vi "ADIS16448 Loop.vi"(8 "error in":errorcluster) -> ()   [LabVIEW 2019]
uses:
  Typedef/ADIS16448 Device Reference.ctl
  Typedef/ADIS16448 Hardware Configuration.ctl
  <vilib>/Rock Robotics/WPI/SPI/WPI_SPIMode.ctl
  <vilib>/Rock Robotics/SystemInterfaces/DIO/FPGA_DIOChannel.ctl
  <vilib>/Rock Robotics/SystemInterfaces/spilib/spi_bus.ctl
  Typedef/ADIS16448 Status.ctl
  Typedef/ADIS16448 Data.ctl
  Typedef/ADIS16448 Process.ctl
  Typedef/ADIS16448 Command Type.ctl
  <vilib>/Rock Robotics/SystemInterfaces/CounterEncoderSourceConvertion/FPGA_CounterEncoderSourceConvertionLVSourceType.ctl
  <vilib>/Rock Robotics/SystemInterfaces/DIO/FPGA_DIODigitalSourceChannel.ctl
  <vilib>/Rock Robotics/SystemInterfaces/AnalogTrigger/FPGA_AnalogTriggerIndex.ctl
  <vilib>/Rock Robotics/SystemInterfaces/AnalogTrigger/FPGA_AnalogTriggerOutType.ctl
  <vilib>/Rock Robotics/WPI/SPI/WPI_SPIDevRef.ctl
  Typedef/ADIS16448 Register.ctl
  <vilib>/Rock Robotics/WPI/Counter/WPI_CounterDigitalInputToDigitalSource.vi
  <vilib>/ptbypt/NI_PtbyPt.lvlib
panel:
  in  "Calibration Time":i32
  in  "element":T1
  in  "ADIS16448DevRef":T2={"DevStatus"={"status"=FALSE, "code"=0, "source"=""}, "Hardware Config"={"SPI Clock Rate (Hz)"=1000000.0, "IMU SPI Mode (3)"=enum."Mode 3 (Clk Idle High,Sample on Trailing)", "IMU Reset Pin"=enum."SPI Port CS2", "IMU SPI Bus"=enum."SPI On-Board, CS0", "IMU Data Ready Pin"=enum."SPI Port CS1", "Stall Config"={"Pow2BytesPerRead"=255, "StallTicks"=640, "CsToSclkTicks"=5}, "IMU Status LED Pin"=enum."DIO MXP 9"}, "Calibration Complete"=refnum, "Status FIFO"=refnum, "Last Value Reference"=refnum, "Sychronous Process VI"=refnum, "Cmd FIFO"=refnum, "Source"={"DevStatus"={"status"=FALSE, "code"=0, "source"=""}, "AnalogTriggerMode?"=FALSE, "DigitalMode"={"DIO Channel"=enum."Disabled"}, "AnalogTriggerMode"={"AnalogTriggerIndex"=enum."Trig 0", "OutputType"=enum."InWindow"}}, "Data FIFO"=refnum, "IMU Status LED Pin"=enum."DIO MXP 9", "Calibration Time"=5}
  in  "Main Name":string
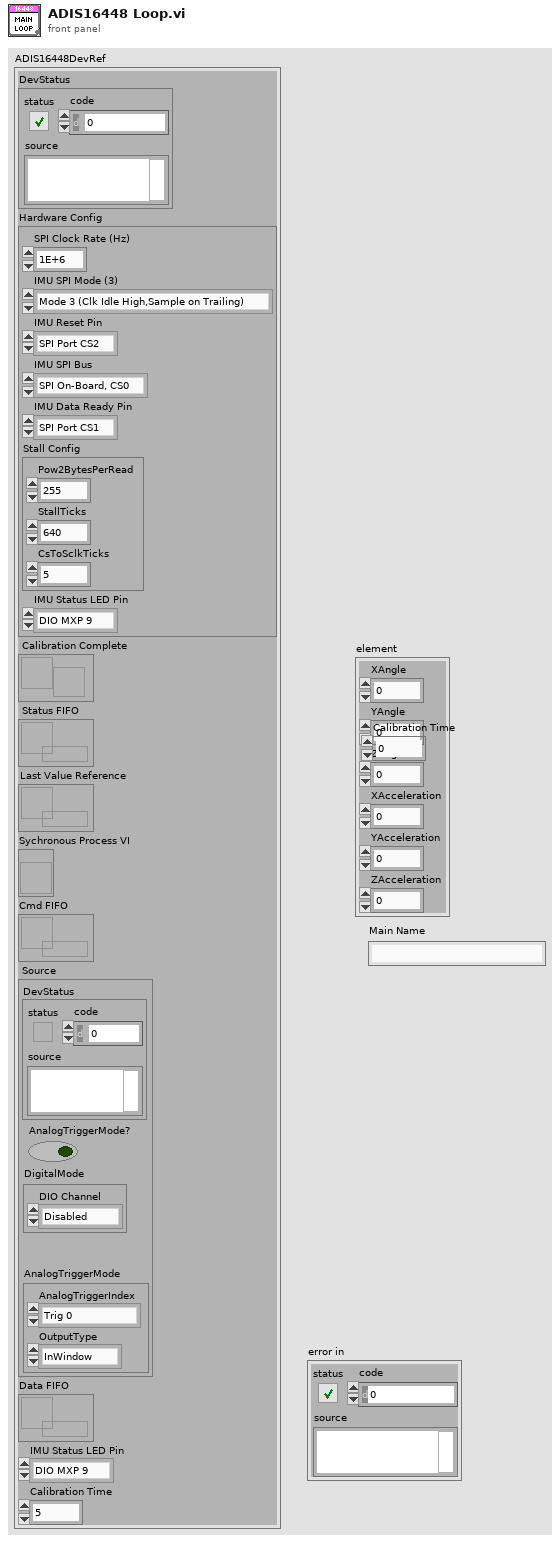
[diagram p1: front panel]
types:
  T1 = typedef "ADIS16448 Data.ctl" = cluster{"XAngle":dbl, "YAngle":dbl, "ZAngle":dbl, "XAcceleration":dbl, "YAcceleration":dbl, "ZAcceleration":dbl}
  T2 = typedef "ADIS16448 Device Reference.ctl" = cluster{"DevStatus":errorcluster, "Hardware Config":T3, "Calibration Complete":refnum<notifier>, "Status FIFO":refnum<k33>, "Last Value Reference":refnum<data-value>, "Sychronous Process VI":T7, "Cmd FIFO":refnum<k33>, "Source":T8, "Data FIFO":refnum<k33>, "IMU Status LED Pin":T5, "Calibration Time":u32}
  T3 = typedef "ADIS16448 Hardware Configuration.ctl" = cluster{"SPI Clock Rate (Hz)":dbl, "IMU SPI Mode (3)":T4, "IMU Reset Pin":T5, "IMU SPI Bus":T6, "IMU Data Ready Pin":T5, "Stall Config":cluster{"Pow2BytesPerRead":u8, "StallTicks":u16, "CsToSclkTicks":u8}, "IMU Status LED Pin":T5}
  T4 = typedef "WPI_SPIMode.ctl" = enum16{"Mode 0 (Clk Idle Low,Sample on Leading)", "Mode 1 (Clk Idle Low,Sample on Trailing)", "Mode 2 (Clk Idle High,Sample on Leading)", "Mode 3 (Clk Idle High,Sample on Trailing)"}
  T5 = typedef "FPGA_DIOChannel.ctl" = enum8{"DIO 0", "DIO 1", "DIO 2", "DIO 3", "DIO 4", "DIO 5", "DIO 6", "DIO 7", "DIO 8", "DIO 9", "DIO MXP 0", "DIO MXP 1", "DIO MXP 2", "DIO MXP 3", "DIO MXP 4", "DIO MXP 5", "DIO MXP 6", "DIO MXP 7", "DIO MXP 8", "DIO MXP 9", "DIO MXP 10", "DIO MXP 11", "DIO MXP 12", "DIO MXP 13", "DIO MXP 14", "DIO MXP 15", "SPI Port CS1", "SPI Port CS2", "SPI Port CS3", "SPI Port MISO", "SPI Port MOSI", "Invalid"}
  T6 = typedef "spi_bus.ctl" = enum16{"SPI On-Board, CS0", "SPI On-Board, CS1", "SPI On-Board, CS2", "SPI On-Board, CS3", "SPI MXP", "Invalid"}
  T7 = typedef "ADIS16448 Process.ctl" = refnum<vi>
  T8 = typedef "FPGA_CounterEncoderSourceConvertionLVSourceType.ctl" = cluster{"DevStatus":errorcluster, "AnalogTriggerMode?":bool, "DigitalMode":cluster{"DIO Channel":T9}, "AnalogTriggerMode":cluster{"AnalogTriggerIndex":T10, "OutputType":T11}}
  T9 = typedef "FPGA_DIODigitalSourceChannel.ctl" = enum8{"DIO 0", "DIO 1", "DIO 2", "DIO 3", "DIO 4", "DIO 5", "DIO 6", "DIO 7", "DIO 8", "DIO 9", "DIO MXP 0", "DIO MXP 1", "DIO MXP 2", "DIO MXP 3", "DIO MXP 4", "DIO MXP 5", "DIO MXP 6", "DIO MXP 7", "DIO MXP 8", "DIO MXP 9", "DIO MXP 10", "DIO MXP 11", "DIO MXP 12", "DIO MXP 13", "DIO MXP 14", "DIO MXP 15", "SPI Port CS1", "SPI Port CS2", "SPI Port CS3", "SPI Port MISO", "SPI Port MOSI", "Disabled"}
  T10 = typedef "FPGA_AnalogTriggerIndex.ctl" = enum8{"Trig 0", "Trig 1", "Trig 2", "Trig 3", "Trig 4", "Trig 5", "Trig 6", "Trig 7", "Invalid"}
  T11 = typedef "FPGA_AnalogTriggerOutType.ctl" = enum16{"InWindow", "TriggerState", "Rising", "Falling"}
  T12 = typedef "WPI_SPIDevRef.ctl" = cluster{"DevStatus":errorcluster, "Handle":i32, "SPI Bus":T6}
  T13 = cluster{"SPIDevRef":T12, "Data Counter":u16, "Reset":bool, "Digital Source":T8, "Bytes Per Sample":u32, "Data":dbl[], "ADIS16448DevRef":T2, "TimeStampPrev":u32, "Sensor to Robot Rotation":dbl[][], "AutoSPI Active?":bool, "Offsets":dbl[], "Offset Counter":i32, "Data Header":u8[], "Zero Byte Count":u8, "Running Offset":dbl[]}
  T14 = typedef "ADIS16448 Status.ctl" = cluster{"Calibrated?":bool, "IMU Detected?":bool}
  T15 = typedef "ADIS16448 Register.ctl" = u8
  T16 = typedef "ADIS16448 Command Type.ctl" = cluster{"Command":enum16{"None", "Reset", "Rewrite Config", "Start Recal", "Recalibrate", "Recal Complete", "Exit Auto SPI", "Start Auto SPI", "Configure Cal"}, "Data":u32}
  T17 = typedef "WPI_DigitalOutputDevRef.ctl" = cluster{"DIO Channel":T5, "DevStatus":errorcluster}
  T18 = typedef "WPI_DigitalInputDevRef.ctl" = cluster{"DevStatus":errorcluster, "DIO Channel":T5}
  T19 = cluster{"Pow2BytesPerRead":u8, "StallTicks":u16, "CsToSclkTicks":u8}
  T20 = enum16{"None", "Reset", "Rewrite Config", "Start Recal", "Recalibrate", "Recal Complete", "Exit Auto SPI", "Start Auto SPI", "Configure Cal"}
  T21 = enum32{"Bad", "Idle", "Run top level", "Running"}
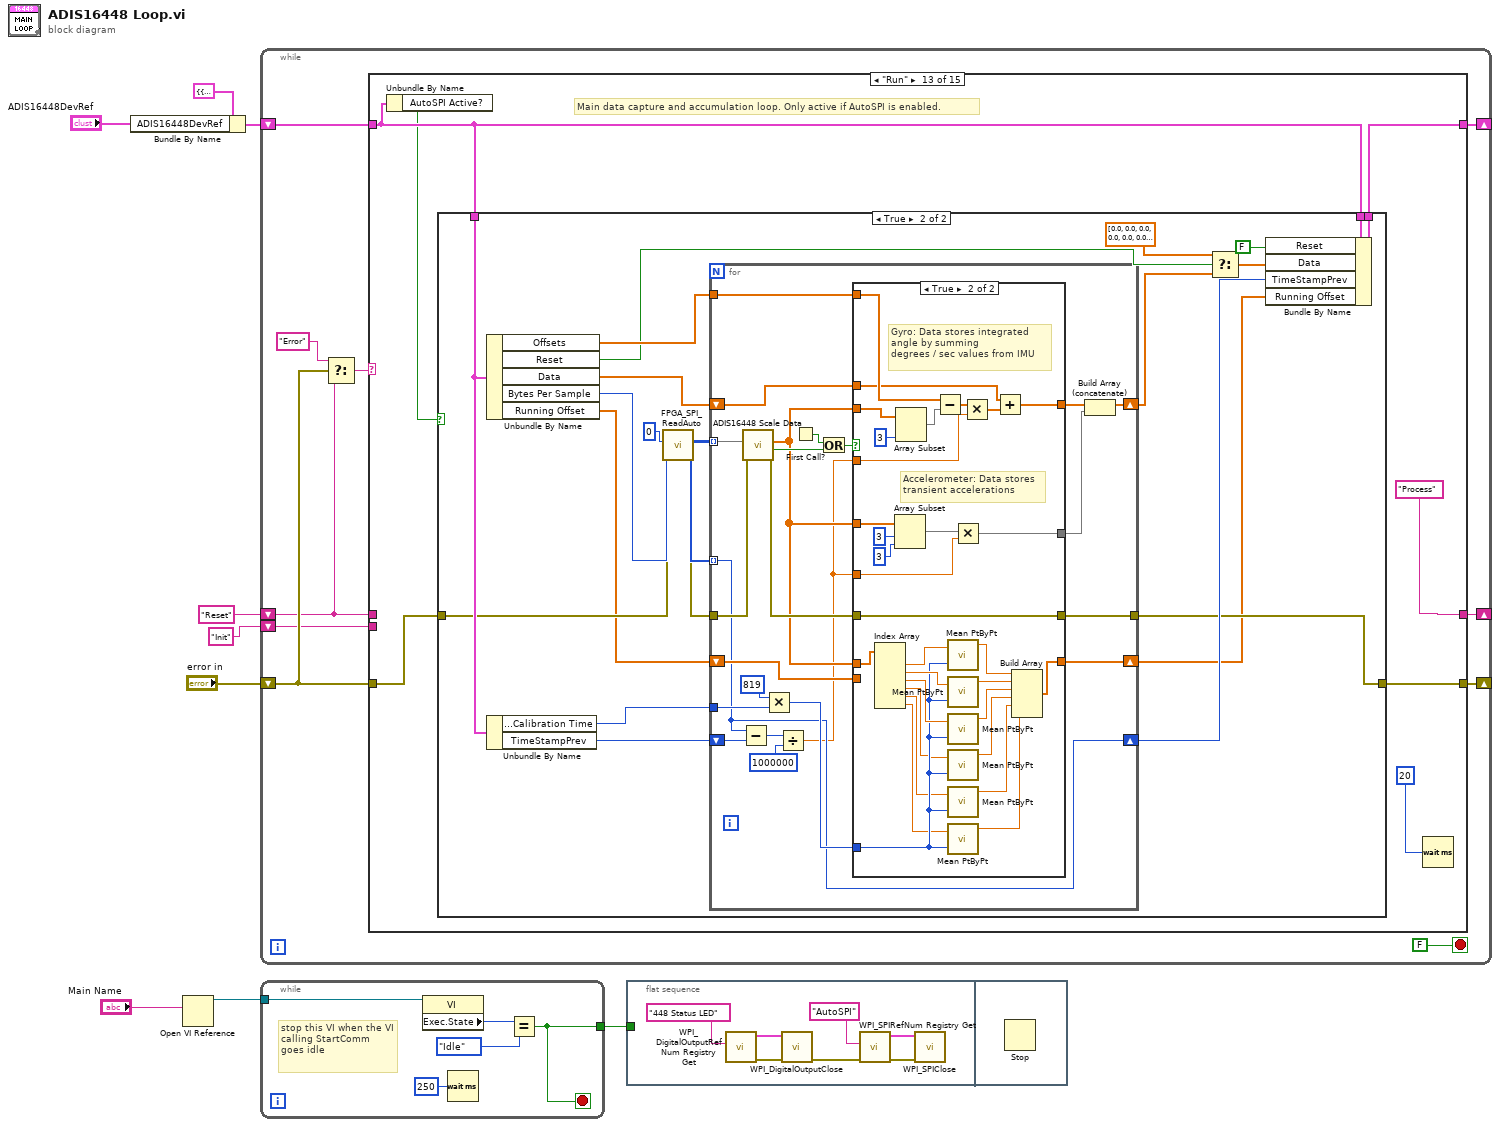
[diagram p0: block diagram]
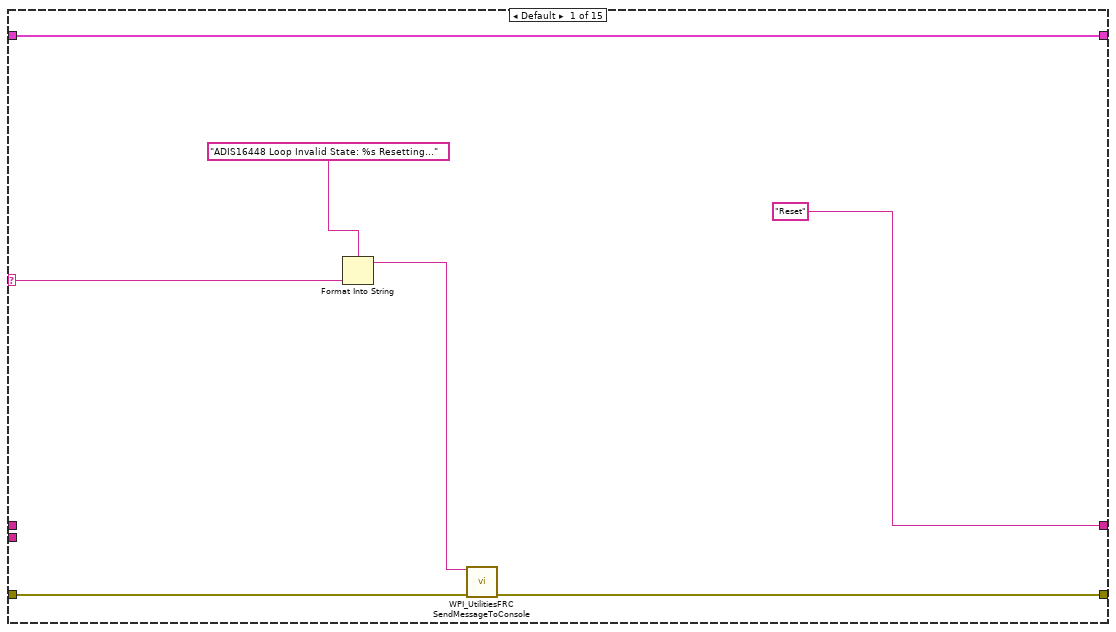
[diagram p2: hidden frame]
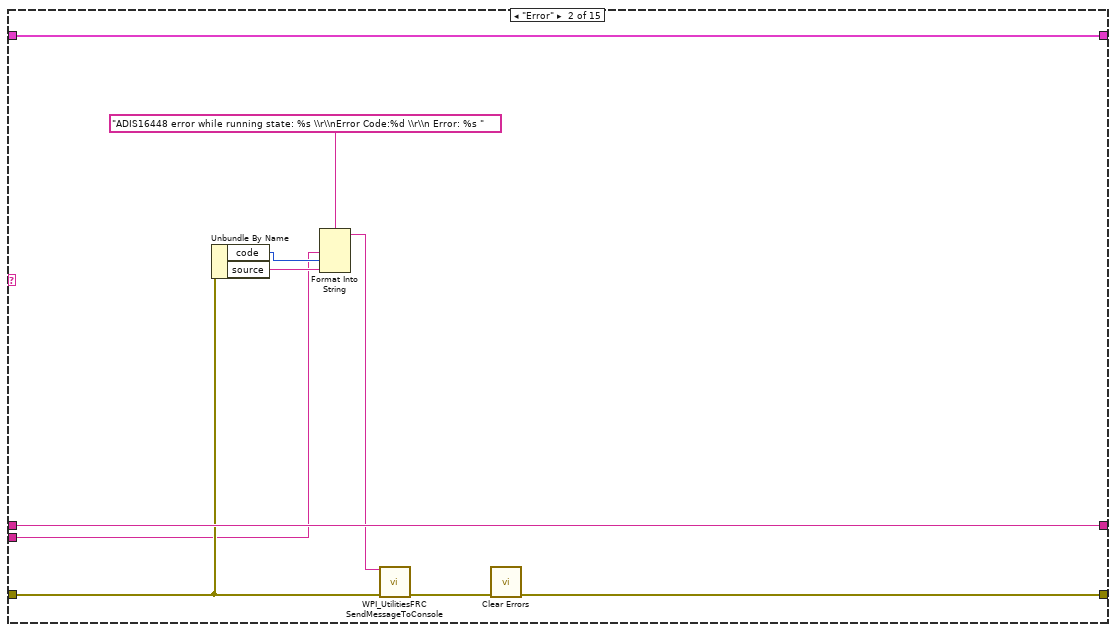
[diagram p3: hidden frame]
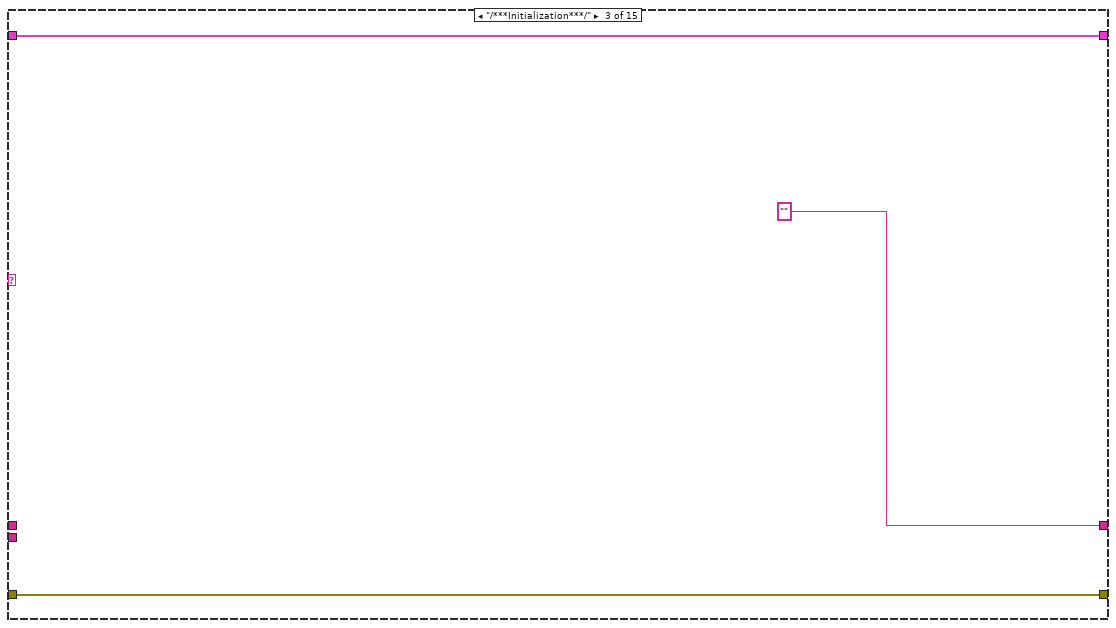
[diagram p4: hidden frame]
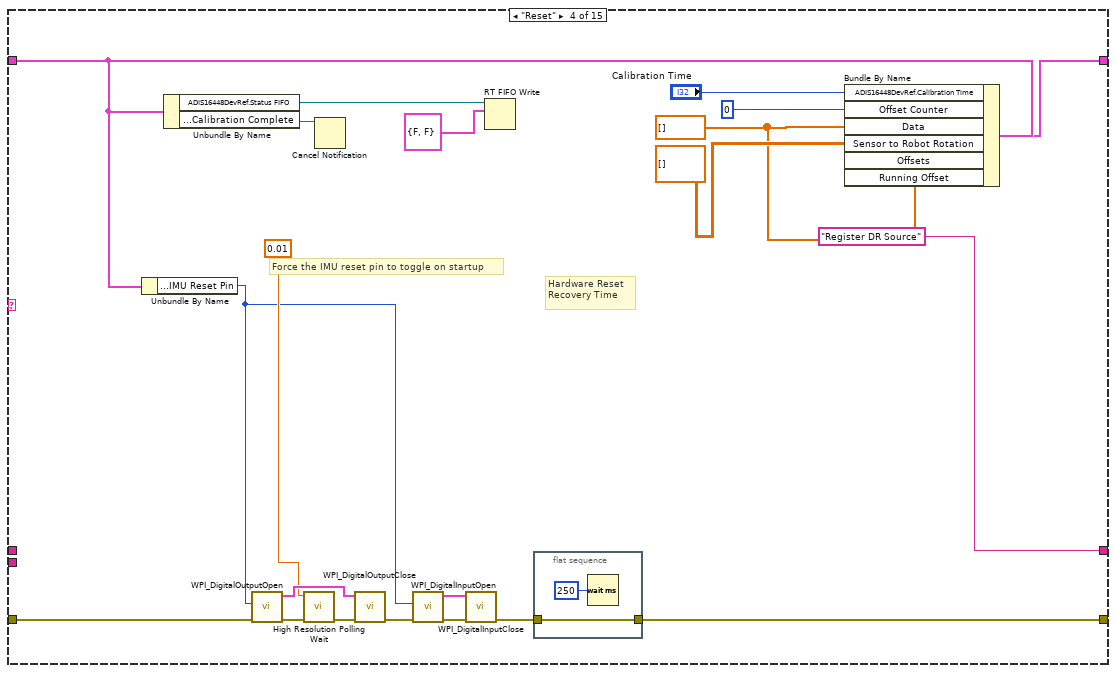
[diagram p5: hidden frame]
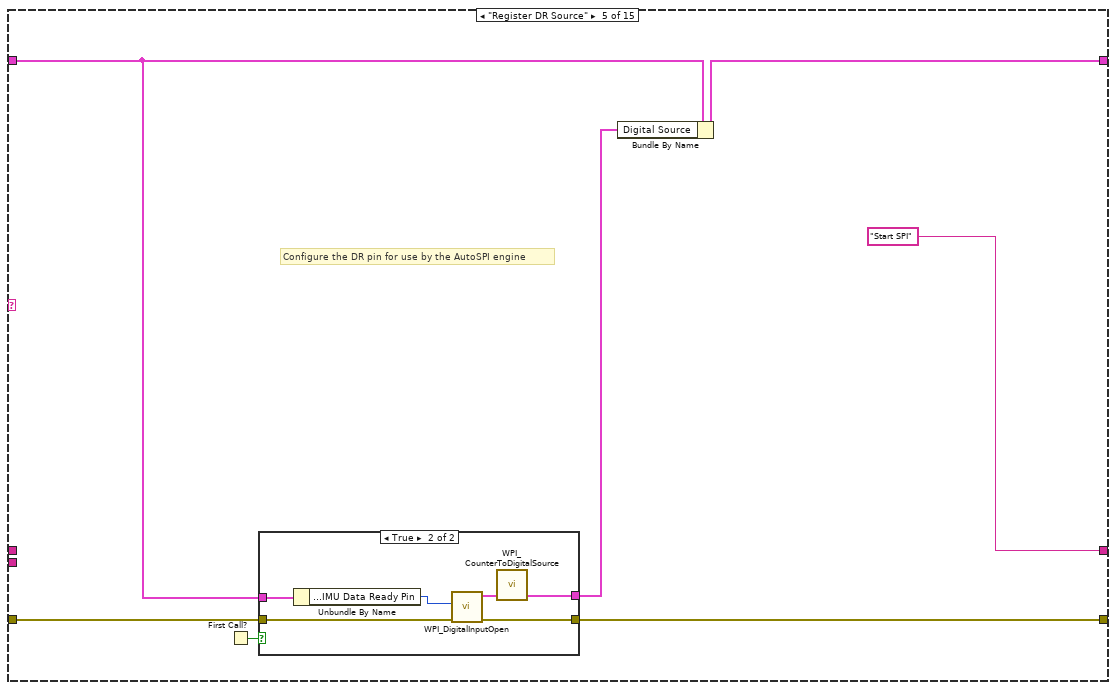
[diagram p6: hidden frame]
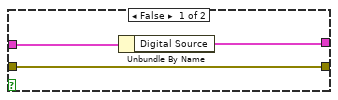
[diagram p7: hidden frame]
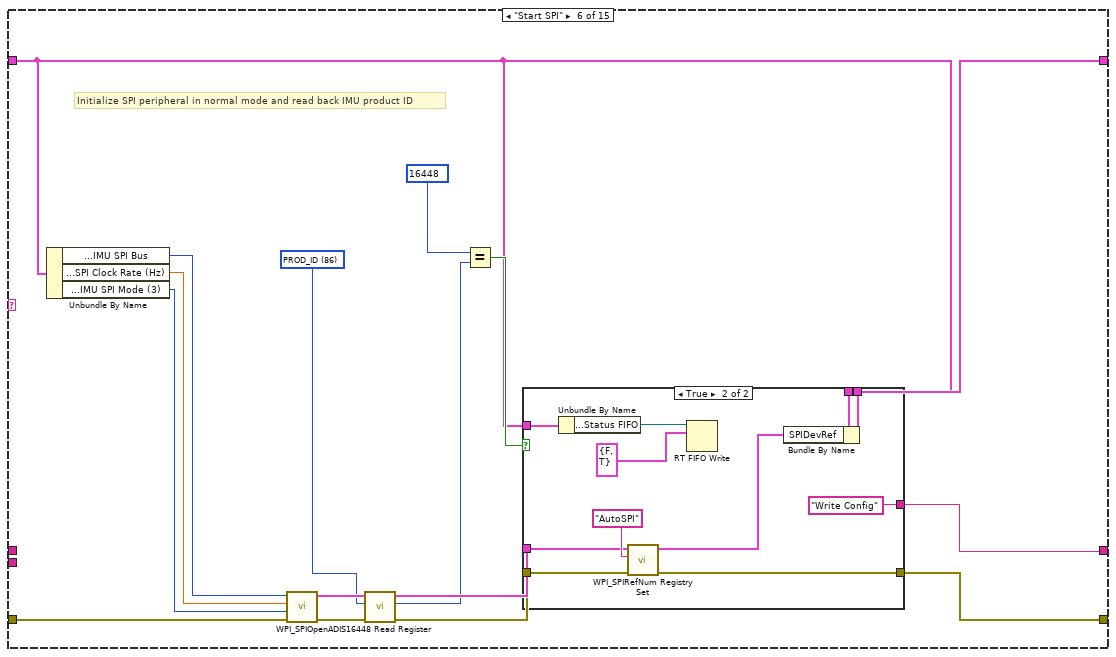
[diagram p8: hidden frame]
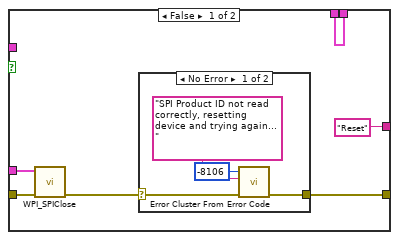
[diagram p9: hidden frame]
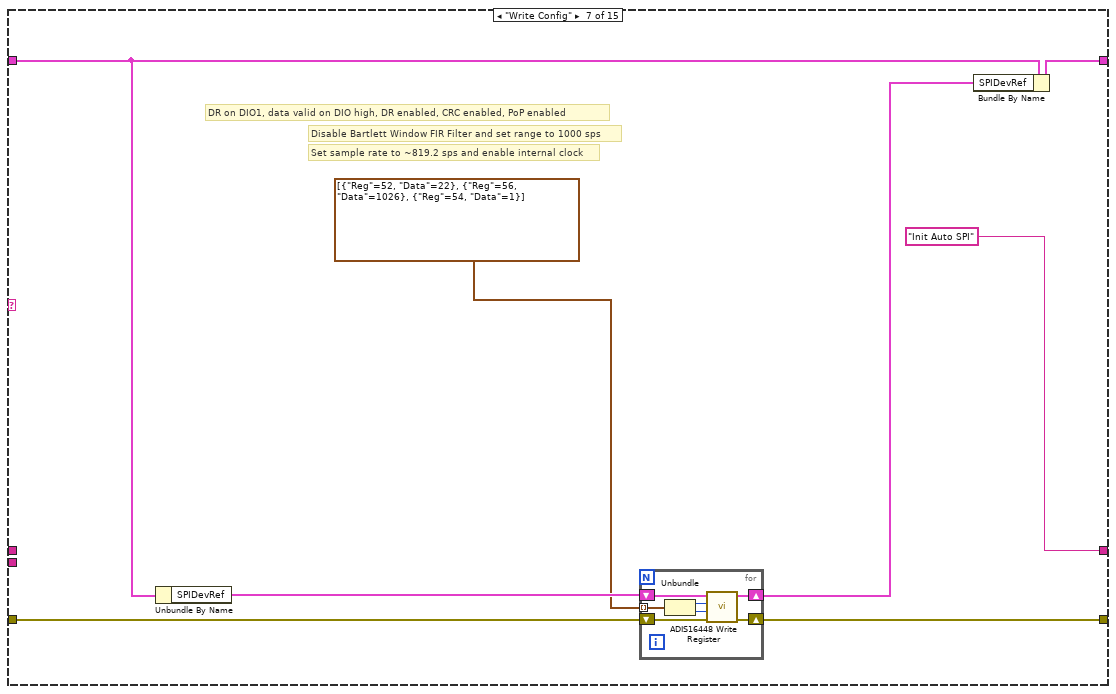
[diagram p11: hidden frame]
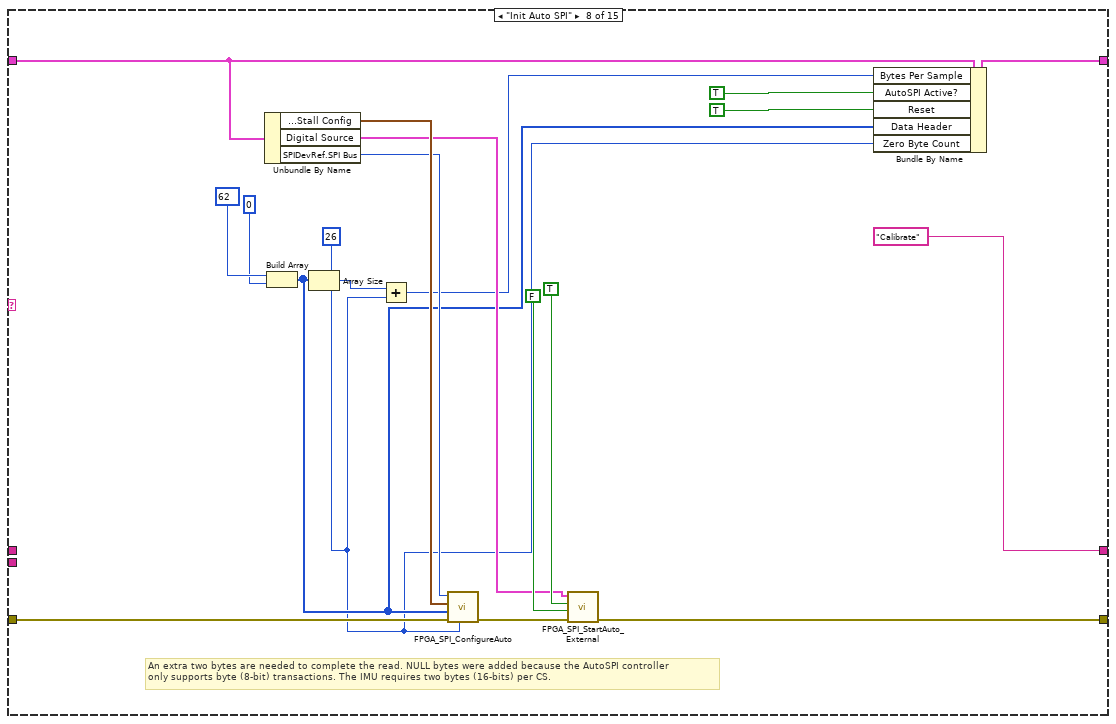
[diagram p12: hidden frame]
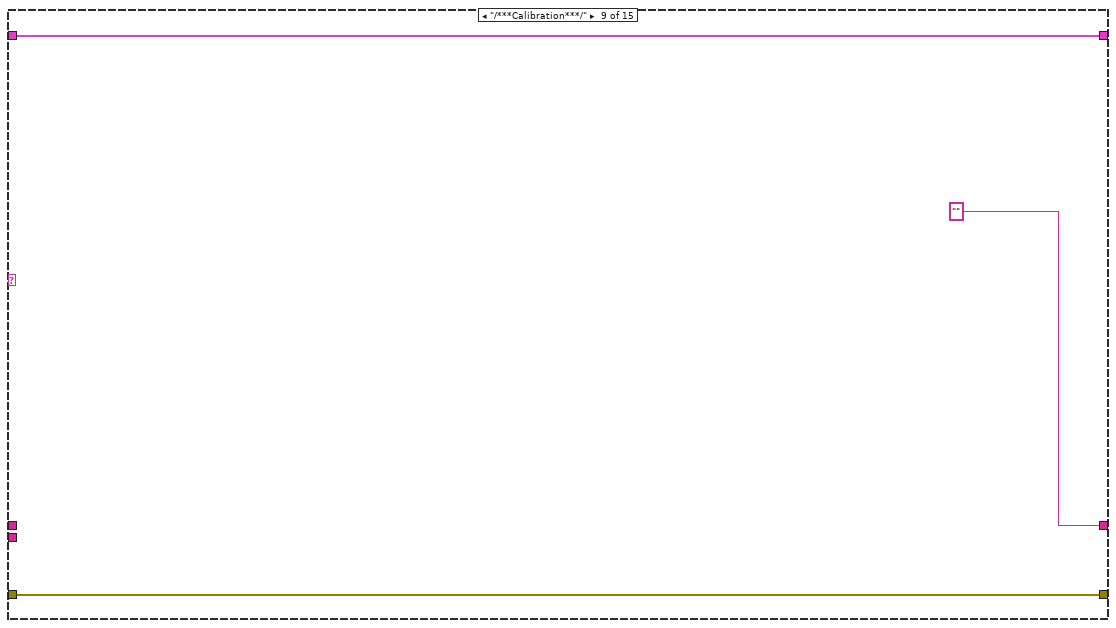
[diagram p13: hidden frame]
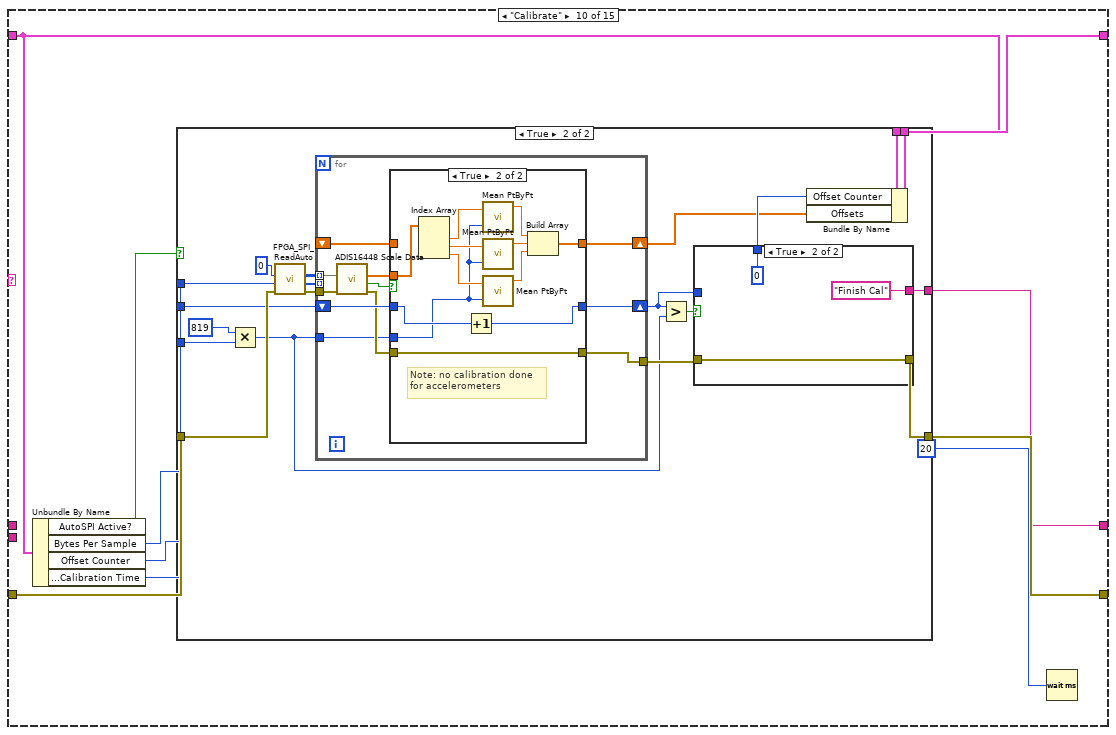
[diagram p14: hidden frame]
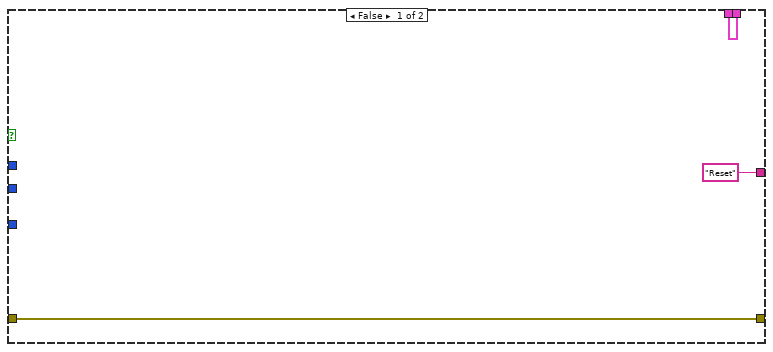
[diagram p15: hidden frame]
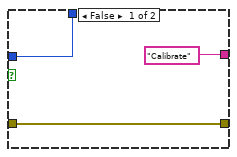
[diagram p16: hidden frame]
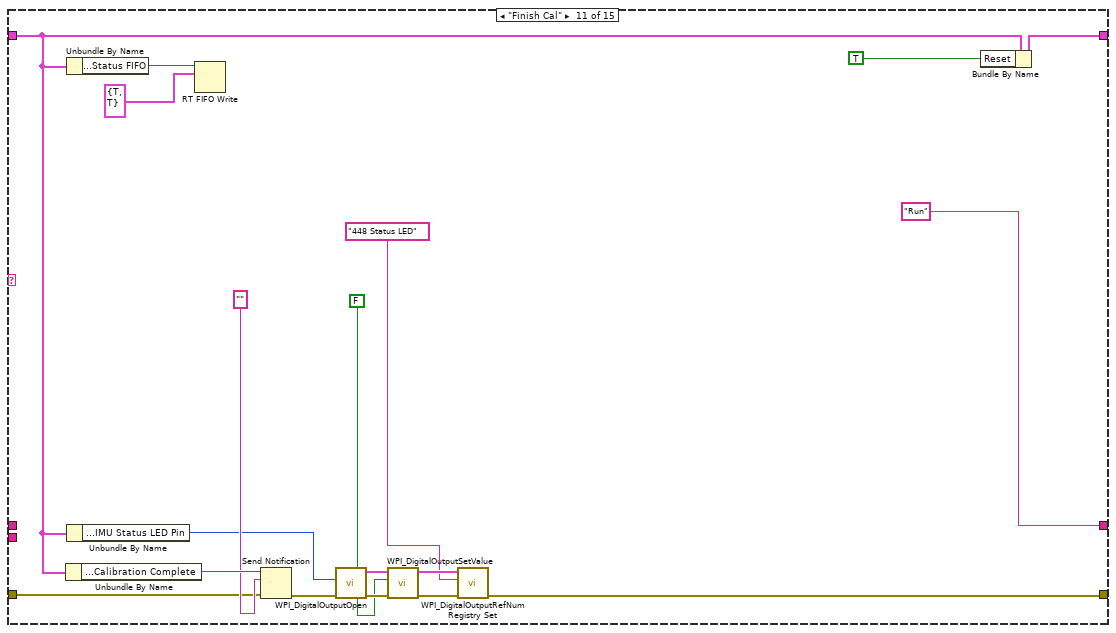
[diagram p18: hidden frame]
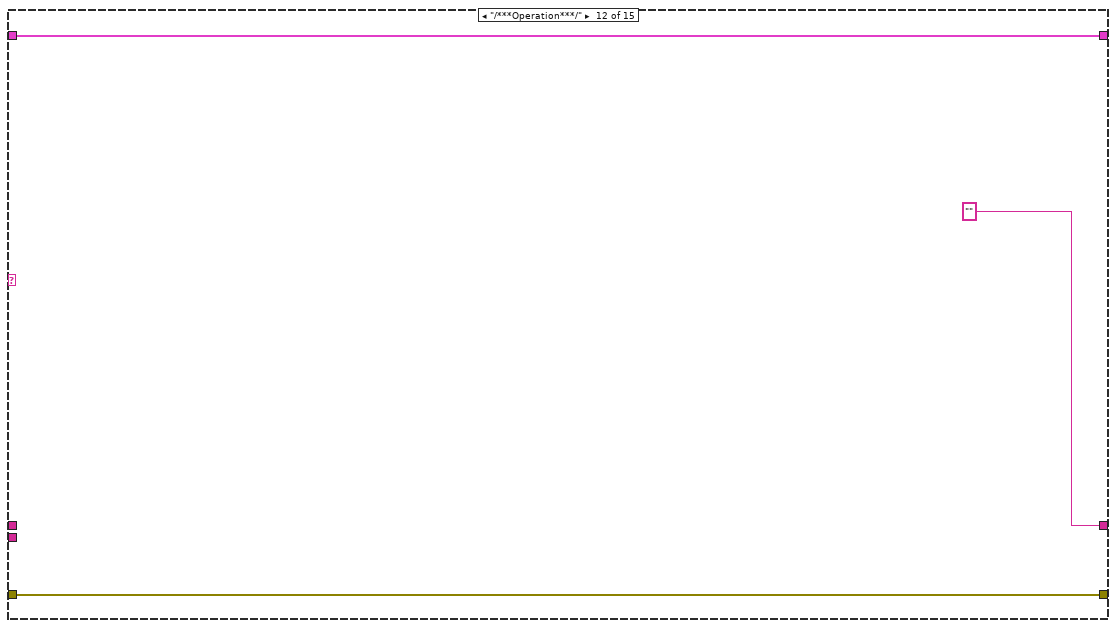
[diagram p19: hidden frame]
diagram:
  n1 = Bundle By Name(cluster=T13 {"SPIDevRef"={"DevStatus"={"status"=FALSE, "code"=0, "source"=""}, "Handle"=0, "SPI Bus"=enum."SPI On-Board, CS0"}, "Data Counter"=0, "Reset"=FALSE, "Digital Source"={"DevStatus"={"status"=FALSE, "code"=0, "source"=""}, "AnalogTriggerMode?"=FALSE, "DigitalMode"={"DIO Channel"=enum."DIO 1"}, "AnalogTriggerMode"={"AnalogTriggerIndex"=enum."Trig 0", "OutputType"=enum."InWindow"}}, "Bytes Per Sample"=0, "Data"=[0.0, 0.0, 0.0, 0.0, 0.0, 0.0, 0.0, 0.0], "ADIS16448DevRef"={"DevStatus"={"status"=FALSE, "code"=0, "source"=""}, "Hardware Config"={"SPI Clock Rate (Hz)"=1000000.0, "IMU SPI Mode (3)"=enum."Mode 3 (Clk Idle High,Sample on Trailing)", "IMU Reset Pin"=enum."SPI Port CS2", "IMU SPI Bus"=enum."SPI On-Board, CS0", "IMU Data Ready Pin"=enum."SPI Port CS1", "Stall Config"={"Pow2BytesPerRead"=255, "StallTicks"=640, "CsToSclkTicks"=5}, "IMU Status LED Pin"=enum."DIO MXP 9"}, "Calibration Complete"=refnum, "Status FIFO"=refnum, "Last Value Reference"=refnum, "Sychronous Process VI"=refnum, "Cmd FIFO"=refnum, "Source"={"DevStatus"={"status"=FALSE, "code"=0, "source"=""}, "AnalogTriggerMode?"=FALSE, "DigitalMode"={"DIO Channel"=enum."Disabled"}, "AnalogTriggerMode"={"AnalogTriggerIndex"=enum."Trig 0", "OutputType"=enum."InWindow"}}, "Data FIFO"=refnum, "IMU Status LED Pin"=enum."DIO MXP 9", "Calibration Time"=5}, "TimeStampPrev"=0, "Sensor to Robot Rotation"=[], "AutoSPI Active?"=TRUE, "Offsets"=[0.0, 0.0, 0.0, 0.0, 0.0, 0.0, 0.0, 0.0], "Offset Counter"=0, "Data Header"=[], "Zero Byte Count"=0, "Running Offset"=[0.0, 0.0, 0.0, 0.0, 0.0, 0.0, 0.0, 0.0]}, "ADIS16448DevRef"="ADIS16448DevRef") -> (w5:T13)
  n2 = Open VI Reference(vi path="Main Name") -> (vi reference=w8:refnum<vi>)  [unwired: 3 in, 3 out]
  n3 = while {
    shift-right: [w15] -> _
    shift-left: "Reset" -> [w12]
    shift-right: [w17] -> _
    shift-left: w5 -> [w18]
    shift-right: [w16] -> _
    shift-left: "error in" -> [w14]
    shift-left: "Init" -> [w10]
    stop <- FALSE stop-if-true
    n4 = Select(t="Error", s=w14, f=w12) -> (s? t:f=w13:string)
    n5 = case shown="\"Run\"" w13 {
      selector: w13 -> [w25 _ _ _ _ _ _ _ _ _ _ _ _ _ _]
      tunnel: w18 -> [w26 w36 w39 w55 w64 w83 w119 w145 w153 w155 w227 w238 w240 w342 w352]
      tunnel: [w26 w36 w39 w54 w68 w88 w118 w144 w153 w160 w234 w238 w244 w342 w358] -> w17
      tunnel: w14 -> [w24 w32 w38 w48 w67 w94 w122 w149 w152 w162 w228 w237 w243 w340 w360]
      tunnel: [w23 w33 w38 w59 w65 w87 w121 w132 w152 w161 w220 w237 w242 w339 w359] -> w16
      tunnel: ["Reset" w35 "" "Register DR Source" "Start SPI" w89 "Init Auto SPI" "Calibrate" "" w156 "Run" "" "Process" "Run Cmds" w350] -> w15
      tunnel: w12 -> [_ w35 _ _ _ _ _ _ _ _ _ _ _ _ _]
      tunnel: w10 -> [_ w27 _ _ _ _ _ _ _ _ _ _ _ _ _]
      frame Default {
        n6 = Format Into String(format string="ADIS16448 Loop Invalid State: %s Resetting...", w25) -> (resulting string=w22:string)  [unwired: 2 in, 1 out]
        n7 = call <vilib>:"WPI_UtilitiesFRC SendMessageToConsole.vi"("Message"=w22, "error in (no error)"=w24) -> ("error out"=w23:errorcluster)  [unwired: 13 in]
      }
      frame "Error" {
        n8 = Unbundle By Name(w32) -> ("code"=w29:i32, "source"=w28:string)
        n9 = Format Into String(format string="ADIS16448 error while running state: %s \\r\\nError Code:%d \\r\\n Error: %s ", w27, w29, w28) -> (resulting string=w31:string)  [unwired: 2 in, 1 out]
        n10 = call <vilib>:"WPI_UtilitiesFRC SendMessageToConsole.vi"("Message"=w31, "error in (no error)"=w32) -> ("error out"=w34:errorcluster)  [unwired: 13 in]
        n11 = call <vilib>:"Clear Errors.vi"("error in (no error)"=w34) -> ("error out"=w33:errorcluster)  [unwired: 5 in, 1 out]
      }
      frame "/***Initialization***/" {
      }
      frame "Reset" {
        w40 = dbl[] [] ("Data")
        # "Hardware Reset Recovery Time"
        # "Force the IMU reset pin to toggle on startup"
        n12 = Unbundle By Name(w55) -> ("ADIS16448DevRef.Hardware Config.IMU Reset Pin"=w44:T5)
        n13 = Unbundle By Name(w55) -> ("ADIS16448DevRef.Status FIFO"=w57:refnum<k33>, "ADIS16448DevRef.Calibration Complete"=w58:refnum<notifier>)
        n14 = call <vilib>:"WPI_DigitalOutputOpen.vi"("error in (no error)"=w48, "DIO Channel"=w44) -> ("error out"=w46:errorcluster, "DigitalOutputDevRef"=w53:T17)  [unwired: 8 in]
        n15 = call <vilib>:"High Resolution Polling Wait.vi"("error in (no error)"=w46, "seconds to wait"=0.01) -> ("error out"=w47:errorcluster)  [unwired: 9 in]
        n16 = Cancel Notification(0:w58) -> ()  [unwired: 1 in, 3 out]
        n17 = call <vilib>:"WPI_DigitalOutputClose.vi"("error in (no error)"=w47, "DigitalOutputDevRef"=w53) -> ("error out"=w50:errorcluster)  [unwired: 9 in]
        n18 = call <vilib>:"WPI_DigitalInputOpen.vi"("error in (no error)"=w50, "DIO Channel"=w44) -> ("error out"=w51:errorcluster, "DigitalInputDevRef"=w52:T18)  [unwired: 8 in]
        n19 = call <vilib>:"WPI_DigitalInputClose.vi"("error in (no error)"=w51, "DigitalInputDevRef"=w52) -> ("error out"=w49:errorcluster)  [unwired: 9 in]
        n20 = RT FIFO Write(0:w57, 1:T14 {"Calibrated?"=FALSE, "IMU Detected?"=FALSE} ("element")) -> ()  [unwired: 3 in, 4 out]
        n21 = flat-sequence {
          tunnel: [w62] -> w59
          tunnel: w49 -> [w62]
          frame #0 {
            n22 = Wait (ms)(milliseconds to wait=u32 250) -> ()  [unwired: 1 out]
          }
        }
        n23 = Bundle By Name(cluster=w55, "ADIS16448DevRef.Calibration Time"="Calibration Time", "Offset Counter"=0, "Data"=w40, "Sensor to Robot Rotation"=dbl[][] [], "Offsets"=w40, "Running Offset"=w40) -> (w54:T13)
      }
      frame "Register DR Source" {
        # "Configure the DR pin for use by the AutoSPI engine"
        n24 = First Call?() -> (First Call?: T/F=w63:bool)
        n25 = case shown="True" w63 {
          tunnel: w67 -> [w70 w78]
          tunnel: w64 -> [w72 w76]
          tunnel: [w71 w74] -> w66
          tunnel: [w70 w73] -> w65
          frame False {
            n26 = Unbundle By Name(w72) -> ("Digital Source"=w71:T8)
          }
          frame True {
            n27 = Unbundle By Name(w76) -> ("ADIS16448DevRef.Hardware Config.IMU Data Ready Pin"=w75:T5)
            n28 = call <vilib>:"WPI_DigitalInputOpen.vi"("error in (no error)"=w78, "DIO Channel"=w75) -> ("error out"=w73:errorcluster, "DigitalInputDevRef"=w77:T18)  [unwired: 8 in]
            n29 = call-poly <vilib>:"WPI_CounterToDigitalSource.vi"("DigitalInputDevRef"=w77) -> ("Digital Source"=w74:T8)  [unwired: 6 in]
          }
        }
        n30 = Bundle By Name(cluster=w64, "Digital Source"=w66) -> (w68:T13)
      }
      frame "Start SPI" {
        w82 = T15 86 items=["FLASH_CNT"=0, "Reserved 1"=2, "XGYRO_OUT"=4, "YGYRO_OUT"=6, "ZGYRO_OUT"=8, "XACCL_OUT"=10, "YACCL_OUT"=12, "ZACCL_OUT"=14, "XMAGN_OUT"=16, "YMAGN_OUT"=18, "ZMAGN_OUT"=20, "BARO_OUT"=22, "TEMP_OUT"=24, "XGYRO_OFF"=26, "YGYRO_OFF"=28, "ZGYRO_OFF"=30, "XACCL_OFF"=32, "YACCL_OFF"=34, "ZACCL_OFF"=36, "XMAGN_HIC"=38, "YMAGN_HIC"=40, "ZMAGN_HIC"=42, "XMAGN_SIC"=44, "YMAGN_SIC"=46, "ZMAGN_SIC"=48, "GPIO_CTRL"=50, "MSC_CTRL"=52, "SMPL_PRD"=54, "SENS_AVG"=56, "SEQ_CNT"=58, "DIAG_STAT"=60, "GLOB_CMD"=62, "ALM_MAG1"=64, "ALM_MAG2"=66, "ALM_SMPL1"=68, "ALM_SMPL2"=70, "ALM_CTRL"=72, "Reserved 2"=74, "Reserved 3"=76, "Reserved 4"=78, "Reserved 5"=80, "LOT_ID1"=82, "LOT_ID2"=84, "PROD_ID"=86, "SERIAL_NUM"=88] ("ADIS16448 Register")
        # "Initialize SPI peripheral in normal mode and read back IMU product ID"
        n31 = Unbundle By Name(w83) -> ("ADIS16448DevRef.Hardware Config.IMU SPI Bus"=w90:T6, "ADIS16448DevRef.Hardware Config.SPI Clock Rate (Hz)"=w91:dbl, "ADIS16448DevRef.Hardware Config.IMU SPI Mode (3)"=w92:T4)
        n32 = call <vilib>:"WPI_SPIOpen.vi"("error in"=w94, "Mode (3)"=w92, "Clock Rate (Hz)"=w91, "SPI Bus"=w90) -> ("error out"=w86:errorcluster, "SPIDevRef"=w85:T12)  [unwired: 6 in]
        n33 = call "ADIS16448 Read Register.vi"("error in (no error)"=w86, "ADIS16448 Register"=w82, "SPIDevRef in"=w85) -> ("error out"=w80:errorcluster, "Register Value"=w79:u16, "SPIDevRef out"=w81:T12)  [unwired: 6 in]
        n34 = Equal?(x=u16 16448 ("y"), y=w79) -> (x = y?=w93:bool)
        n35 = case shown="True" w93 {
          tunnel: ["Reset" "Write Config"] -> w89
          tunnel: w83 -> [w99 w115]
          tunnel: [w99 w114] -> w88
          tunnel: [w98 w109] -> w87
          tunnel: w80 -> [w97 w110]
          tunnel: w81 -> [w96 w111]
          tunnel: w83 -> [_ w106]
          frame False {
            n36 = call <vilib>:"WPI_SPIClose.vi"("error in (no error)"=w97, "SPIDevRef"=w96) -> ("error out"=w95:errorcluster)  [unwired: 9 in]
            n37 = case shown="No Error" w95 {
              selector: w95 -> [w103 w105]
              tunnel: [w104 w105] -> w98
              frame No Error {
                n38 = call <vilib>:"Error Cluster From Error Code.vi"("error in (no error)"=w103, "error message (\"\")"="SPI Product ID not read correctly, resetting device and trying again..." ("error message (\"\")"), "error code (0)"=-8106) -> ("error out"=w104:errorcluster)  [unwired: 6 in]
              }
              frame Error {
              }
            }
          }
          frame True {
            n39 = Unbundle By Name(w106) -> ("ADIS16448DevRef.Status FIFO"=w108:refnum<k33>)
            n40 = call <vilib>:"WPI_SPIRefNum Registry Set.vi"("error in (no error)"=w110, "refnum name"="AutoSPI", "SPIDevRef"=w111) -> ("error out"=w109:errorcluster, "SPIDevRef"=w113:T12)  [unwired: 7 in]
            n41 = RT FIFO Write(0:w108, 1:T14 {"Calibrated?"=FALSE, "IMU Detected?"=TRUE} ("element")) -> ()  [unwired: 3 in, 4 out]
            n42 = Bundle By Name(cluster=w115, "SPIDevRef"=w113) -> (w114:T13)
          }
        }
      }
      frame "Write Config" {
        # "DR on DIO1, data valid on DIO high, DR enabled, CRC enabled, PoP enabled"
        # "Set sample rate to ~819.2 sps and enable internal clock"
        # "Disable Bartlett Window FIR Filter and set range to 1000 sps"
        n43 = Unbundle By Name(w119) -> ("SPIDevRef"=w123:T12)
        n44 = for {
          tunnel: cluster{"Reg":T15, "Data":u16}[] [{"Reg"=52, "Data"=22}, {"Reg"=56, "Data"=1026}, {"Reg"=54, "Data"=1}] -> [w131] mode=indexing
          shift-right: [w127] -> w121
          shift-left: w122 -> [w126]
          shift-right: [w125] -> w117
          shift-left: w123 -> [w128]
          n45 = Unbundle(w131) -> ("Reg"=w130:T15, "Data"=w129:u16)
          n46 = call "ADIS16448 Write Register.vi"("error in (no error)"=w126, "Data"=w129, "Register"=w130, "SPIDevRef in"=w128) -> ("error out"=w127:errorcluster, "SPIDevRef out"=w125:T12)  [unwired: 6 in]
        }
        n47 = Bundle By Name(cluster=w119, "SPIDevRef"=w117) -> (w118:T13)
      }
      frame "Init Auto SPI" {
        w133 = u8 26 ("dimension size")
        # "An extra two bytes are needed to complete the read. NULL bytes were added because the AutoSPI controller \nonly supports byte (8-bit) transactions. The IMU requires two bytes (16-bits) per CS."
        n48 = Unbundle By Name(w145) -> ("ADIS16448DevRef.Hardware Config.Stall Config"=w143:T19, "Digital Source"=w141:T8, "SPIDevRef.SPI Bus"=w140:T6)
        n49 = Build Array(u8 62 ("hi"), u8 0 ("element")) -> (w134:u8[])
        n50 = Array Size(array=w134) -> (size(s)=w138:i32)
        n51 = Add(x=w138, y=w133) -> (x+y=w135:i32)
        n52 = call <vilib>:"FPGA_SPI_ConfigureAuto.vi"("SPI Auto Zero Byte Count"=w133, "error in"=w149, "SPI Auto TX Byte Array"=w134, "Stall Config"=w143, "SPI Bus"=w140) -> ("error out"=w148:errorcluster)  [unwired: 6 in]
        n53 = call <vilib>:"FPGA_SPI_StartAuto_External.vi"("error in (no error)"=w148, "Falling Edge"=FALSE, "Rising Edge"=TRUE, "Source"=w141) -> ("error out"=w132:errorcluster)  [unwired: 7 in]
        n54 = Bundle By Name(cluster=w145, "Bytes Per Sample"=w135, "AutoSPI Active?"=TRUE, "Reset"=TRUE, "Data Header"=w134, "Zero Byte Count"=w133) -> (w144:T13)
      }
      frame "/***Calibration***/" {
      }
      frame "Calibrate" {
        n55 = Unbundle By Name(w155) -> ("AutoSPI Active?"=w163:bool, "Bytes Per Sample"=w159:u32, "Offset Counter"=w158:i32, "ADIS16448DevRef.Calibration Time"=w157:u32)
        n56 = case shown="True" w163 {
          tunnel: [w166 w185] -> w160
          tunnel: w162 -> [w165 w180]
          tunnel: [w165 w170] -> w161
          tunnel: w155 -> [w166 w181]
          tunnel: w159 -> [_ w178]
          tunnel: w158 -> [_ w175]
          tunnel: w157 -> [_ w176]
          tunnel: ["Reset" w171] -> w156
          frame False {
          }
          frame True {
            n57 = Multiply(x=819, y=w176) -> (x*y=w167:u32)
            n58 = call <vilib>:"FPGA_SPI_ReadAuto.vi"("error in (no error)"=w180, "Bytes per Sample"=w178, "Samples to Read"=u32 0) -> ("error out"=w179:errorcluster, "Timestamps"=w182:u32[], "Data"=w183:u8[][])  [unwired: 6 in]
            n59 = for {
              tunnel: w183 -> [w202] mode=indexing
              tunnel: w182 -> [_] mode=indexing
              tunnel: w179 -> [w201]
              tunnel: [w196] -> w169
              shift-right: [w197] -> w173
              shift-left: w175 -> [w198]
              shift-right: [w194] -> w168
              shift-left: _ -> [w193]
              tunnel: w167 -> [w192]
              n60 = call "ADIS16448 Scale Data.vi"("error in (no error)"=w201, "New Data In"=w202) -> ("error out"=w195:errorcluster, "Data Good?"=w200:bool, "Data Out"=w199:dbl[])  [unwired: 7 in]
              n61 = case shown="True" w200 {
                tunnel: w199 -> [_ w211]
                tunnel: w198 -> [w205 w208]
                tunnel: [w205 w207] -> w197
                tunnel: [w204 w209] -> w196
                tunnel: w195 -> [w204 w209]
                tunnel: [w203 w210] -> w194
                tunnel: w193 -> [w203 _]
                tunnel: w192 -> [_ w206]
                frame False {
                }
                frame True {
                  # "Note: no calibration done\nfor accelerometers"
                  n62 = Index Array(array=w211) -> (element #1=w212:dbl, element #2=w213:dbl, element #3=w214:dbl)  [unwired: 3 in]
                  n63 = Increment(x=w208) -> (x+1=w207:i32)
                  n64 = call <vilib>:"Mean PtByPt.vi"("x"=w212, "sample length"=w206) -> ("mean"=w215:dbl)  [unwired: 2 in, 1 out]
                  n65 = call <vilib>:"Mean PtByPt.vi"("x"=w213, "sample length"=w206) -> ("mean"=w216:dbl)  [unwired: 2 in, 1 out]
                  n66 = call <vilib>:"Mean PtByPt.vi"("x"=w214, "sample length"=w206) -> ("mean"=w217:dbl)  [unwired: 2 in, 1 out]
                  n67 = Build Array(w215, w216, w217) -> (w210:dbl[])
                }
              }
            }
            n68 = Greater?(x=w173, y=w167) -> (0:w174:bool)
            n69 = case shown="True" w174 {
              tunnel: w173 -> [w188 _]
              tunnel: [w188 u32 0 ("Offset Counter")] -> w172
              tunnel: ["Calibrate" "Finish Cal"] -> w171
              tunnel: [w186 w189] -> w170
              tunnel: w169 -> [w186 w189]
              frame False {
              }
              frame True {
              }
            }
            n70 = Bundle By Name(cluster=w181, "Offset Counter"=w172, "Offsets"=w168) -> (w185:T13)
          }
        }
        n71 = Wait (ms)(milliseconds to wait=u32 20) -> ()  [unwired: 1 out]
      }
      frame "Finish Cal" {
        n72 = Unbundle By Name(w227) -> ("ADIS16448DevRef.Calibration Complete"=w232:refnum<notifier>)
        n73 = Unbundle By Name(w227) -> ("ADIS16448DevRef.Status FIFO"=w230:refnum<k33>)
        n74 = Unbundle By Name(w227) -> ("ADIS16448DevRef.Hardware Config.IMU Status LED Pin"=w218:T5)
        n75 = RT FIFO Write(0:w230, 1:T14 {"Calibrated?"=TRUE, "IMU Detected?"=TRUE} ("element")) -> ()  [unwired: 3 in, 4 out]
        n76 = Send Notification(notification="", notifier=w232, error in (no error)=w228) -> (error out=w221:errorcluster)  [unwired: 1 out]
        n77 = call <vilib>:"WPI_DigitalOutputOpen.vi"("error in (no error)"=w221, "DIO Channel"=w218) -> ("error out"=w226:errorcluster, "DigitalOutputDevRef"=w225:T17)  [unwired: 8 in]
        n78 = call <vilib>:"WPI_DigitalOutputSetValue.vi"("error in (no error)"=w226, "Value"=FALSE, "DigitalOutputDevRef"=w225) -> ("error out"=w224:errorcluster, "DigitalOutputDevRef"=w223:T17)  [unwired: 7 in]
        n79 = call <vilib>:"WPI_DigitalOutputRefNum Registry Set.vi"("error in (no error)"=w224, "refnum name"="448 Status LED", "DigitalOutputDevRef"=w223) -> ("error out"=w220:errorcluster)  [unwired: 7 in, 1 out]
        n80 = Bundle By Name(cluster=w227, "Reset"=TRUE ("First Run")) -> (w234:T13)
      }
      frame "/***Operation***/" {
      }
      frame "Run" {
        # "Main data capture and accumulation loop. Only active if AutoSPI is enabled."
        n81 = Unbundle By Name(w240) -> ("AutoSPI Active?"=w239:bool)
        n82 = case shown="True" w239 {
          tunnel: [w247 w269] -> w244
          tunnel: w243 -> [w246 w256]
          tunnel: [w246 w253] -> w242
          tunnel: w240 -> [w247 w260]
          tunnel: w240 -> [_ w257]
          frame False {
          }
          frame True {
            n83 = Unbundle By Name(w257) -> ("Offsets"=w254:dbl[], "Reset"=w252:bool, "Data"=w263:dbl[], "Bytes Per Sample"=w267:u32, "Running Offset"=w250:dbl[])
            n84 = Unbundle By Name(w257) -> ("ADIS16448DevRef.Calibration Time"=w251:u32, "TimeStampPrev"=w259:u32)
            n85 = call <vilib>:"FPGA_SPI_ReadAuto.vi"("error in (no error)"=w256, "Bytes per Sample"=w267, "Samples to Read"=u32 0) -> ("error out"=w255:errorcluster, "Timestamps"=w264:u32[], "Data"=w265:u8[][])  [unwired: 6 in]
            n86 = for {
              tunnel: w265 -> [w291] mode=indexing
              tunnel: w264 -> [w275] mode=indexing
              shift-right: [w270] -> w248
              shift-left: w263 -> [w286]
              shift-right: [w275] -> w258
              shift-left: w259 -> [w292]
              tunnel: w255 -> [w290]
              tunnel: w254 -> [w289]
              tunnel: [w284] -> w253
              tunnel: w251 -> [w280]
              shift-right: [w276] -> w249
              shift-left: w250 -> [w277]
              n87 = Subtract(x=w275, y=w292) -> (x-y=w288:u32)
              n88 = call "ADIS16448 Scale Data.vi"("error in (no error)"=w290, "New Data In"=w291) -> ("error out"=w285:errorcluster, "Data Good?"=w282:bool, "Data Out"=w274:dbl[])  [unwired: 7 in]
              n89 = Multiply(x=819, y=w280) -> (x*y=w278:u32)
              n90 = Divide(x=w288, y=u32 1000000) -> (x/y=w273:dbl)
              n91 = First Call?() -> (First Call?: T/F=w281:bool)
              n92 = Or(x=w281, y=w282) -> (x .or. y?=w283:bool)
              n93 = case shown="True" w283 {
                tunnel: w274 -> [_ w329]
                tunnel: w289 -> [_ w327]
                tunnel: w273 -> [_ w325]
                tunnel: [w296 w324] -> w272
                tunnel: w286 -> [w293 w322]
                tunnel: w285 -> [w299 w321]
                tunnel: [w299 w321] -> w284
                tunnel: w274 -> [_ w314]
                tunnel: w278 -> [_ w312]
                tunnel: w277 -> [w298 _]
                tunnel: [w298 w313] -> w276
                tunnel: w274 -> [_ w305]
                tunnel: w273 -> [_ w301]
                tunnel: [w294 w300] -> w271
                frame False {
                  w295 = 3 ("length")
                  n94 = Array Subset(array=w293, length=3) -> (w296:dbl[])  [unwired: 1 in]
                  n95 = Array Subset(array=w293, index=w295, length=w295) -> (w294:dbl[])
                }
                frame True {
                  # "Accelerometer: Data stores\ntransient accelerations"
                  # "Gyro: Data stores integrated\nangle by summing\ndegrees / sec values from IMU"
                  n96 = Index Array(array=w314) -> (element #1=w315:dbl, element #2=w316:dbl, element #3=w317:dbl, element #4=w309:dbl, element #5=w310:dbl, element #6=w311:dbl)  [unwired: 6 in]
                  n97 = Array Subset(array=w305, index=3, length=3) -> (w302:dbl[])
                  n98 = Array Subset(array=w329, length=3) -> (w328:dbl[])  [unwired: 1 in]
                  n99 = Subtract(x=w327, y=w328) -> (x-y=w326:dbl[])
                  n100 = call <vilib>:"Mean PtByPt.vi"("x"=w315, "sample length"=w312) -> ("mean"=w318:dbl)  [unwired: 2 in, 1 out]
                  n101 = call <vilib>:"Mean PtByPt.vi"("x"=w316, "sample length"=w312) -> ("mean"=w319:dbl)  [unwired: 2 in, 1 out]
                  n102 = call <vilib>:"Mean PtByPt.vi"("x"=w317, "sample length"=w312) -> ("mean"=w320:dbl)  [unwired: 2 in, 1 out]
                  n103 = call <vilib>:"Mean PtByPt.vi"("x"=w309, "sample length"=w312) -> ("mean"=w308:dbl)  [unwired: 2 in, 1 out]
                  n104 = call <vilib>:"Mean PtByPt.vi"("x"=w310, "sample length"=w312) -> ("mean"=w307:dbl)  [unwired: 2 in, 1 out]
                  n105 = call <vilib>:"Mean PtByPt.vi"("x"=w311, "sample length"=w312) -> ("mean"=w306:dbl)  [unwired: 2 in, 1 out]
                  n106 = Multiply(x=w302, y=w301) -> (x*y=w300:dbl[])
                  n107 = Multiply(x=w326, y=w325) -> (x*y=w323:dbl[])
                  n108 = Add(x=w322, y=w323) -> (x+y=w324:dbl[])
                  n109 = Build Array(w318, w319, w320, w308, w307, w306) -> (w313:dbl[])
                }
              }
              n110 = Build Array (concatenate)(w272, w271) -> (w270:dbl[])
            }
            n111 = Select(t=dbl[] [0.0, 0.0, 0.0, 0.0, 0.0, 0.0, 0.0, 0.0] ("Angle and Vel"), s=w252, f=w248) -> (s? t:f=w261:dbl[])
            n112 = Bundle By Name(cluster=w260, "Reset"=FALSE ("First Run"), "Data"=w261, "TimeStampPrev"=w258, "Running Offset"=w249) -> (w269:T13)
          }
        }
        n113 = Wait (ms)(milliseconds to wait=u32 20) -> ()  [unwired: 1 out]
      }
      frame "Process" {
        n114 = Unbundle By Name(w342) -> ("ADIS16448DevRef.Sychronous Process VI"=w337:T7, "ADIS16448DevRef.Data FIFO"=w341:refnum<k33>, "Data"=w336:dbl[])
        n115 = Index Array(array=w336) -> (element #1=w335:dbl, element #2=w334:dbl, element #3=w333:dbl)  [unwired: 3 in]
        n116 = Bundle By Name(cluster="element", "XAngle"=w335, "YAngle"=w334, "ZAngle"=w333) -> (w331:T1)
        n117 = RT FIFO Write(0:w341, 1:w331) -> ()  [unwired: 3 in, 4 out]
        n118 = Not A Number/Path/Refnum?(number/path/refnum=w337) -> (NaN/Path/Refnum?=w338:bool)
        n119 = case shown="False" w338 {
          tunnel: w340 -> [w344 w349]
          tunnel: w331 -> [_ _]
          tunnel: [w348 w349] -> w339
          tunnel: w337 -> [w347 _]
          frame False {
            n120 = call-by-ref "?"(reference=w347, error in=w344, 8:"error in (no error)"=w344) -> (error out=w345:errorcluster, 0:"error out"=w346:errorcluster)  [unwired: 10 in, 1 out]
            n121 = Merge Errors(w345, w346) -> (w348:errorcluster)
          }
          frame True {
          }
        }
      }
      frame "Run Cmds" {
        n122 = Unbundle By Name(w352) -> ("ADIS16448DevRef.Cmd FIFO"=w361:refnum<k33>)
        n123 = Unbundle By Name(w352) -> ("ADIS16448DevRef.Status FIFO"=w356:refnum<k33>, "ADIS16448DevRef.Calibration Complete"=w357:refnum<notifier>)
        n124 = RT FIFO Read(0:w361, 1:T16 {"Command"=enum."None", "Data"=0} ("element")) -> (8:w355:refnum<k33>, 9:w354:T16)  [unwired: 2 in, 3 out]
        n125 = Unbundle(w354) -> ("Command"=w351:T20, "Data"=w353:u32)
        n126 = case shown="\"Exit Auto SPI\"" w351 {
          tunnel: w352 -> [w364 w370 w379 w390 w399 w417 w463 w480 w487]
          tunnel: w360 -> [w365 w369 w377 w387 w404 w433 w473 w483 w488]
          tunnel: [w365 w369 w376 w387 w404 w420 w464 w483 w488] -> w359
          tunnel: [w364 w368 w379 w391 w398 w416 w463 w480 w486] -> w358
          tunnel: w357 -> [_ _ _ _ w403 _ _ _ _]
          tunnel: w356 -> [_ _ _ _ w401 w408 _ w481 _]
          tunnel: w355 -> [_ _ w374 w394 _ w431 w475 w477 _]
          tunnel: w353 -> [_ _ _ _ _ _ _ _ w484]
          tunnel: w352 -> [_ _ w373 w392 _ w414 w462 _ _]
          tunnel: ["Run" "Run" "Run" "Run" "Run" w405 "Run" "Run" "Run"] -> w350
          frame "None", Default {
          }
          frame "Reset" {
            n127 = Bundle By Name(cluster=w370, "Reset"=TRUE ("First Run")) -> (w368:T13)
          }
          frame "Rewrite Config" {
            n128 = Unbundle By Name(w373) -> ("SPIDevRef"=w372:T12)
            n129 = RT FIFO Write(0:w374, 1:T16 {"Command"=enum."Start Auto SPI", "Data"=0} ("element")) -> ()  [unwired: 3 in, 4 out]
            n130 = for {
              tunnel: cluster{"Reg":T15, "Data":u16}[] [{"Reg"=52, "Data"=22}, {"Reg"=56, "Data"=1026}, {"Reg"=54, "Data"=1}] -> [w386] mode=indexing
              shift-right: [w382] -> w376
              shift-left: w377 -> [w381]
              shift-right: [w380] -> _
              shift-left: w372 -> [w383]
              n131 = Unbundle(w386) -> ("Reg"=w385:T15, "Data"=w384:u16)
              n132 = call "ADIS16448 Write Register.vi"("error in (no error)"=w381, "Data"=w384, "Register"=w385, "SPIDevRef in"=w383) -> ("error out"=w382:errorcluster, "SPIDevRef out"=w380:T12)  [unwired: 6 in]
            }
          }
          frame "Recalibrate" {
            n133 = Unbundle By Name(w392) -> ("Running Offset"=w389:dbl[])
            n134 = RT FIFO Write(0:w394, 1:T16 {"Command"=enum."Recal Complete", "Data"=0} ("element")) -> ()  [unwired: 3 in, 4 out]
            n135 = Bundle By Name(cluster=w390, "Offsets"=w389) -> (w391:T13)
          }
          frame "Recal Complete" {
            n136 = Send Notification(notification="", notifier=w403) -> ()  [unwired: 1 in, 2 out]
            n137 = RT FIFO Write(0:w401, 1:T14 {"Calibrated?"=TRUE, "IMU Detected?"=TRUE} ("element")) -> ()  [unwired: 3 in, 4 out]
            n138 = Bundle By Name(cluster=w399, "AutoSPI Active?"=TRUE, "Reset"=TRUE) -> (w398:T13)
          }
          frame "Exit Auto SPI" {
            w427 = T15 114 items=["Reserved1"=0, "DIAG_STAT"=2, "X_GYRO_LOW"=4, "X_GYRO_OUT"=6, "Y_GYRO_LOW"=8, "Y_GYRO_OUT"=10, "Z_GYRO_LOW"=12, "Z_GYRO_OUT"=14, "X_ACCL_LOW"=16, "X_ACCL_OUT"=18, "Y_ACCL_LOW"=20, "Y_ACCL_OUT"=22, "Z_ACCL_LOW"=24, "Z_ACCL_OUT"=26, "TEMP_OUT"=28, "TIME_STAMP"=30, "Reseved2"=32, "DATA_CNTR"=34, "X_DELTANG_LOW"=36, "X_DELTANG_OUT"=38, "Y_DELTANG_LOW"=40, "Y_DELTANG_OUT"=42, "Z_DELTANG_LOW"=44, "Z_DELTANG_OUT"=46, "X_DELTVEL_LOW"=48, "X_DELTVEL_OUT"=50, "Y_DELTVEL_LOW"=52, "Y_DELTVEL_OUT"=54, "Z_DELTVEL_LOW"=56, "Z_DELTVEL_OUT"=58, "Reserved3"=60, "Reserved4"=62, "XG_BIAS_LOW"=64, "XG_BIAS_HIGH"=66, "YG_BIAS_LOW"=68, "YG_BIAS_OUT"=70, "ZG_BIAS_LOW"=72, "ZG_BIAS_OUT"=74, "XA_BIAS_LOW"=76, "XA_BIAS_HIGH"=78, "YA_BIAS_LOW"=80, "YA_BIAS_OUT"=82, "ZA_BIAS_LOW"=84, "ZA_BIAS_OUT"=86, "Reserved5"=88, "Reserved6"=90, "FILT_CTRL"=92, "Reserved5"=94, "MSC_CTRL"=96, "UP_SCALE"=98, "DEC_RATE"=100, "NULL_CNFG"=102, "GLOB_CMD"=104, "Reserved6"=106, "FIRM_REV"=108, "FIRM_DM"=110, "FIRM_Y"=112, "PROD_ID"=114, "SERIAL_NUM"=116, "USER_SCR1"=118, "USER_SCR2"=120, "USER_SCR3"=122, "FLSHCNT_LOW"=124, "FLSHCNT_HIGH"=126] ("ADIS16448 Register")
            n139 = Unbundle By Name(w414) -> ("ADIS16448DevRef.Hardware Config.IMU SPI Bus"=w430:T6, "ADIS16448DevRef.Hardware Config.SPI Clock Rate (Hz)"=w429:dbl, "ADIS16448DevRef.Hardware Config.IMU SPI Mode (3)"=w428:T4, "SPIDevRef"=w409:T12)
            n140 = RT FIFO Write(0:w408, 1:T14 {"Calibrated?"=FALSE, "IMU Detected?"=FALSE} ("element")) -> (8:w406:refnum<k33>)  [unwired: 3 in, 3 out]
            n141 = RT FIFO Write(0:w431, 1:T16 {"Command"=enum."Rewrite Config", "Data"=0} ("element")) -> ()  [unwired: 3 in, 4 out]
            n142 = call <vilib>:"WPI_SPIClose.vi"("error in (no error)"=w433, "SPIDevRef"=w409) -> ("error out"=w418:errorcluster)  [unwired: 9 in]
            n143 = call <vilib>:"WPI_DigitalOutputRefNum Registry Get.vi"("error in (no error)"=w418, "refnum name"="448 Status LED") -> ("error out"=w412:errorcluster, "DigitalOutputDevRef"=w411:T17)  [unwired: 8 in]
            n144 = call <vilib>:"WPI_DigitalOutputSetValue.vi"("error in (no error)"=w412, "Value"=TRUE, "DigitalOutputDevRef"=w411) -> ("error out"=w413:errorcluster)  [unwired: 7 in, 1 out]
            n145 = call <vilib>:"WPI_SPIOpen.vi"("error in"=w413, "Mode (3)"=w428, "Clock Rate (Hz)"=w429, "SPI Bus"=w430) -> ("error out"=w426:errorcluster, "SPIDevRef"=w422:T12)  [unwired: 6 in]
            n146 = call "ADIS16448 Read Register.vi"("error in (no error)"=w426, "ADIS16448 Register"=w427, "SPIDevRef in"=w422) -> ("error out"=w423:errorcluster, "Register Value"=w421:u16, "SPIDevRef out"=w424:T12)  [unwired: 6 in]
            n147 = Equal?(x=u16 16448 ("y"), y=w421) -> (x = y?=w425:bool)
            n148 = case shown="True" w425 {
              tunnel: w424 -> [w436 w453]
              tunnel: w423 -> [w437 w452]
              tunnel: [w439 w451] -> w420
              tunnel: w417 -> [w438 w449]
              tunnel: [w438 w448] -> w416
              tunnel: w406 -> [_ w447]
              tunnel: ["Reset" "Run"] -> w405
              frame False {
                n149 = call <vilib>:"WPI_SPIClose.vi"("error in (no error)"=w437, "SPIDevRef"=w436) -> ("error out"=w435:errorcluster)  [unwired: 9 in]
                n150 = case shown="No Error" w435 {
                  selector: w435 -> [w441 w444]
                  tunnel: [w440 w444] -> w439
                  frame No Error {
                    n151 = call <vilib>:"Error Cluster From Error Code.vi"("error in (no error)"=w441, "error message (\"\")"="SPI port did not reset properly" ("error message (\"\")"), "error code (0)"=-8106) -> ("error out"=w440:errorcluster)  [unwired: 6 in]
                  }
                  frame Error {
                  }
                }
              }
              frame True {
                n152 = call <vilib>:"WPI_SPIRefNum Registry Set.vi"("error in (no error)"=w452, "refnum name"="AutoSPI", "SPIDevRef"=w453) -> ("error out"=w451:errorcluster, "SPIDevRef"=w454:T12)  [unwired: 7 in]
                n153 = RT FIFO Write(0:w447, 1:T14 {"Calibrated?"=FALSE, "IMU Detected?"=TRUE} ("element")) -> ()  [unwired: 3 in, 4 out]
                n154 = Bundle By Name(cluster=w449, "SPIDevRef"=w454, "AutoSPI Active?"=FALSE) -> (w448:T13)
              }
            }
          }
          frame "Start Auto SPI" {
            n155 = Unbundle By Name(w462) -> ("SPIDevRef"=w461:T12, "Digital Source"=w460:T8, "ADIS16448DevRef.Hardware Config.Stall Config"=w459:T19, "Data Header"=w458:u8[], "Zero Byte Count"=w457:u8)
            n156 = Unbundle By Name(w461) -> ("SPI Bus"=w474:T6)
            n157 = RT FIFO Write(0:w475, 1:T16 {"Command"=enum."Recal Complete", "Data"=0} ("element")) -> ()  [unwired: 3 in, 4 out]
            n158 = call <vilib>:"FPGA_SPI_ConfigureAuto.vi"("SPI Auto Zero Byte Count"=w457, "error in"=w473, "SPI Auto TX Byte Array"=w458, "Stall Config"=w459, "SPI Bus"=w474) -> ("error out"=w466:errorcluster)  [unwired: 6 in]
            n159 = call <vilib>:"FPGA_SPI_StartAuto_External.vi"("error in (no error)"=w466, "Falling Edge"=FALSE, "Rising Edge"=TRUE, "Source"=w460) -> ("error out"=w470:errorcluster)  [unwired: 7 in]
            n160 = call <vilib>:"WPI_DigitalOutputRefNum Registry Get.vi"("error in (no error)"=w470, "refnum name"="448 Status LED") -> ("error out"=w469:errorcluster, "DigitalOutputDevRef"=w468:T17)  [unwired: 8 in]
            n161 = call <vilib>:"WPI_DigitalOutputSetValue.vi"("error in (no error)"=w469, "Value"=FALSE, "DigitalOutputDevRef"=w468) -> ("error out"=w464:errorcluster)  [unwired: 7 in, 1 out]
          }
          frame "Start Recal" {
            n162 = RT FIFO Write(0:w481, 1:T14 {"Calibrated?"=FALSE, "IMU Detected?"=TRUE} ("element")) -> ()  [unwired: 3 in, 4 out]
            n163 = RT FIFO Write(0:w477, 1:T16 {"Command"=enum."Recalibrate", "Data"=0} ("element")) -> ()  [unwired: 3 in, 4 out]
          }
          frame "Configure Cal" {
            n164 = Bundle By Name(cluster=w487, "ADIS16448DevRef.Calibration Time"=w484) -> (w486:T13)
          }
        }
      }
    }
  }
  n165 = while {
    tunnel: w8 -> [w490]
    tunnel: [w489] -> w2
    stop <- w489 stop-if-true
    # "stop this VI when the VI calling StartComm goes idle"
    n166 = property class="VI"(reference=w490) -> ("Exec.State"=w492:T21)  [unwired: 1 in, 2 out]
    n167 = Wait (ms)(milliseconds to wait=u32 250) -> ()  [unwired: 1 out]
    n168 = Equal?(x=w492, y=T21."Idle" ("Execution:State")) -> (x = y?=w489:bool)
  }
  n169 = flat-sequence {
    tunnel: w2 -> [_]
    frame #0 {
      n170 = call <vilib>:"WPI_DigitalOutputRefNum Registry Get.vi"("refnum name"="448 Status LED") -> ("error out"=w499:errorcluster, "DigitalOutputDevRef"=w498:T17)  [unwired: 9 in]
      n171 = call <vilib>:"WPI_DigitalOutputClose.vi"("error in (no error)"=w499, "DigitalOutputDevRef"=w498) -> ("error out"=w494:errorcluster)  [unwired: 9 in]
      n172 = call <vilib>:"WPI_SPIRefNum Registry Get.vi"("error in (no error)"=w494, "refnum name"="AutoSPI") -> ("error out"=w496:errorcluster, "SPIDevRef"=w495:T12)  [unwired: 8 in]
      n173 = call <vilib>:"WPI_SPIClose.vi"("error in (no error)"=w496, "SPIDevRef"=w495) -> ()  [unwired: 9 in, 1 out]
    }
    frame #1 {
      n174 = Stop() -> ()  [unwired: 1 in]
    }
  }
